vi "Write Sub Panel Productos.vi"(8 "error in (no error)":errorcluster, 10 "Sub Panel Productos":refnum<vi>, 11 "REFRESCOS Y PAPAS ACTOR in":refnum<class "REFRESCOS Y PAPAS ACTOR.lvclass">) -> (0 "error out":errorcluster, 3 "REFRESCOS Y PAPAS ACTOR out":refnum<class "REFRESCOS Y PAPAS ACTOR.lvclass">)   [LabVIEW 2019, in "REFRESCOS Y PAPAS ACTOR.lvlib" / "REFRESCOS Y PAPAS ACTOR.lvclass"]
uses:
  REFRESCOS Y PAPAS ACTOR.lvclass
  REFRESCOS Y PAPAS ACTOR.lvclass/REFRESCOS Y PAPAS ACTOR.ctl
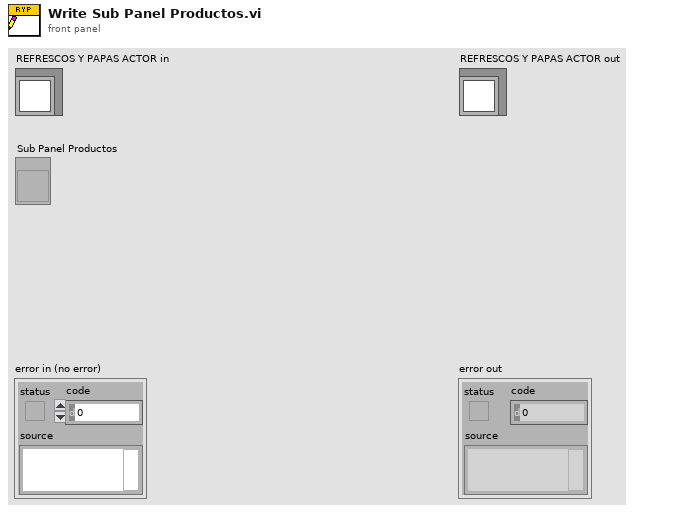
[diagram p1: front panel]
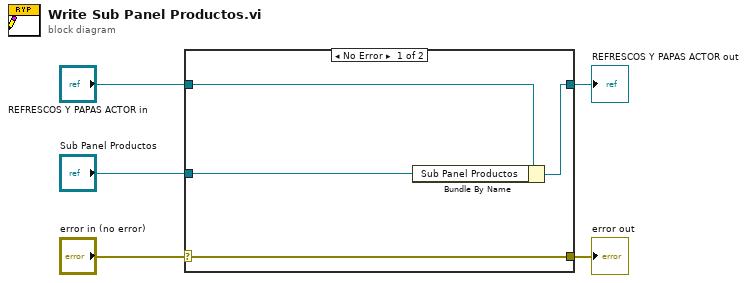
[diagram p0: block diagram]
diagram:
  n1 = case shown="No Error" "error in (no error)" {
    selector: "error in (no error)" -> [w9 w10]
    tunnel: [w9 w10] -> w4
    tunnel: [w7 w11] -> w2
    tunnel: "REFRESCOS Y PAPAS ACTOR in" -> [w8 w11]
    tunnel: "Sub Panel Productos" -> [w6 _]
    frame No Error {
      n2 = Bundle By Name(cluster=w8, "Sub Panel Productos"=w6) -> (w7:refnum<class "REFRESCOS Y PAPAS ACTOR.lvclass">)
    }
    frame Error {
    }
  }
  "error out" <- w4
  "REFRESCOS Y PAPAS ACTOR out" <- w2
